vi "Material-Line 3-Normalize.vi"(8 "error in (no error)":errorcluster, 11 "Material-RunTest in":refnum<class "Material-RunTest.lvclass">) -> (0 "error out":errorcluster, 3 "Material-RunTest out":refnum<class "Material-RunTest.lvclass">)   [LabVIEW 2014, in "Material-RunTest.lvclass"]
uses:
  Material-RunTest.lvclass
  <userlib>/_MGI/1D Array/MGI Average/MGI Average (DBL[]).vi
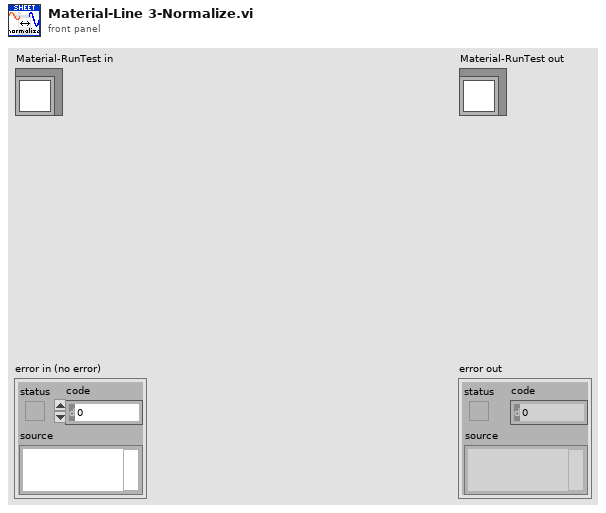
[diagram p1: front panel]
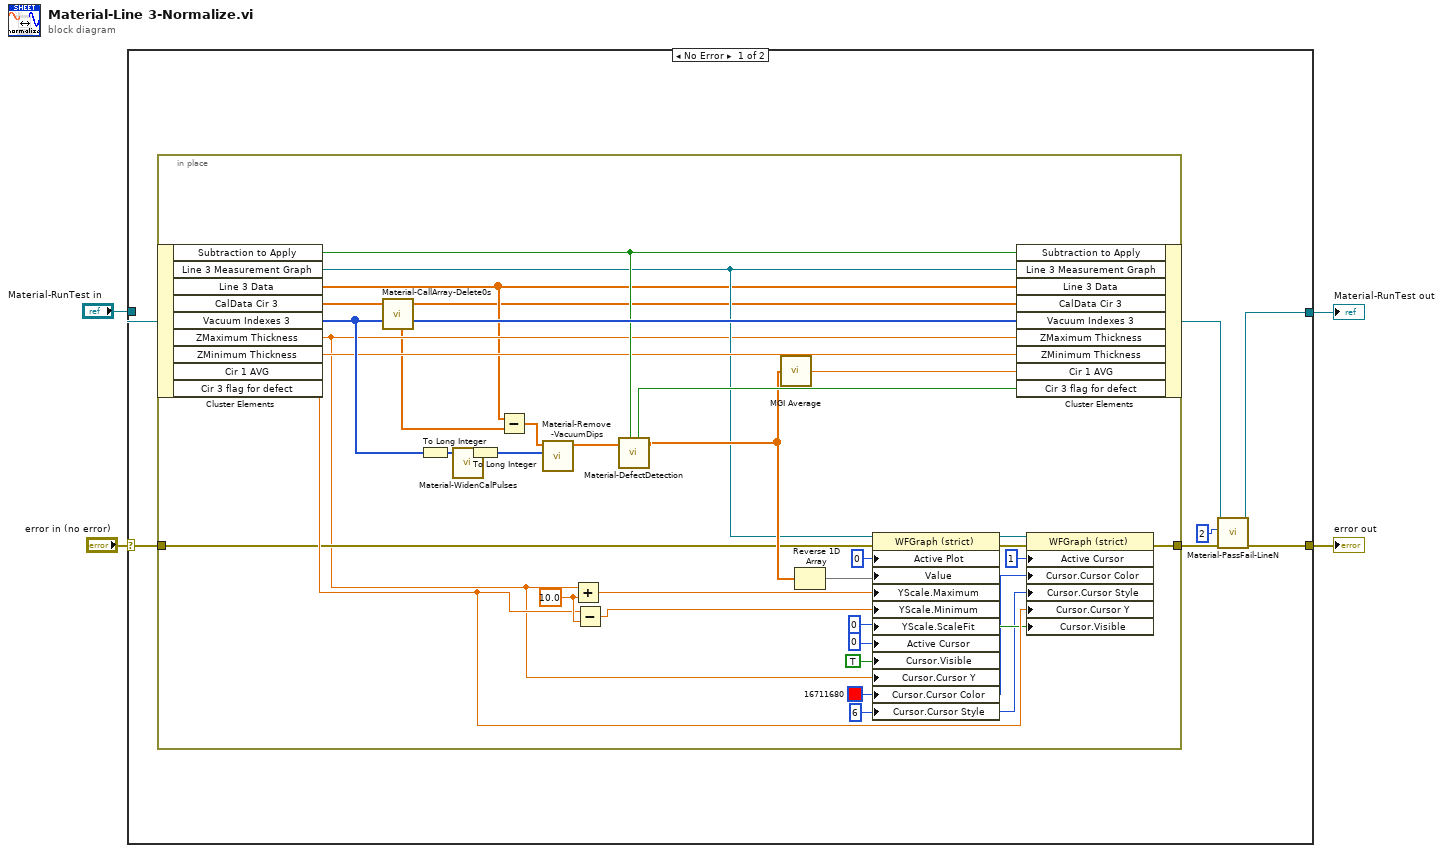
[diagram p0: block diagram]
diagram:
  n1 = case shown="No Error" "error in (no error)" {
    selector: "error in (no error)" -> [w10 w44]
    tunnel: [w7 w44] -> w3
    tunnel: [w5 w43] -> w1
    tunnel: "Material-RunTest in" -> [w11 w43]
    frame No Error {
      n2 = in-place {
        in-place-border: w10 -> [w28]
        in-place-border: [w34] -> w9
        w22 = u32 16711680
        w21 = u8 6 ("Cursor.Cursor Style")
        w23 = TRUE ("Cursor.Visible")
        w38 = 10.0 ("y")
        n3 = in-place-cluster #1(w11) -> ("Subtraction to Apply"=w32:bool, "Line 3 Measurement Graph"=w27:refnum<vi>, "Line 3 Data"=w14:dbl[], "CalData Cir 3"=w13:dbl[], "Vacuum Indexes 3"=w37:i32[], "ZMaximum Thickness"=w20:dbl, "ZMinimum Thickness"=w29:dbl)  [unwired: 2 out]
        n4 = call "Material-CallArray-Delete0s.vi"("CalData Line 3"=w13) -> ("array w/ subset deleted"=w12:dbl[])  [unwired: 8 in]
        n5 = To Long Integer(number=w37) -> (32bit integer=w39:i32[])
        n6 = call "Material-WidenCalPulses.vi"("raw CAL indexes"=w39) -> ("New Indexes"=w41:u32[])  [unwired: 8 in]
        n7 = To Long Integer(number=w41) -> (32bit integer=w42:i32[])
        n8 = Subtract(x=w14, y=w12) -> (x-y=w40:dbl[])
        n9 = call "Material-Remove-VacuumDips.vi"("input array of indexes"=w42, "Input Data"=w40) -> ("Conditioned output"=w33:dbl[])  [unwired: 9 in]
        n10 = Add(x=w20, y=w38) -> (x+y=w18:dbl)
        n11 = Subtract(x=w29, y=w38) -> (x-y=w19:dbl)
        n12 = call "Material-DefectDetection.vi"("Conditioned output"=w33, "Subtraction to Apply"=w32) -> ("Flagged for Defect"=w31:bool, "Array"=w30:dbl[])  [unwired: 6 in]
        n13 = call-poly <userlib>:"MGI Average.vi"("Double[]"=w30) -> ("Average"=w36:dbl)  [unwired: 1 in]
        n14 = Reverse 1D Array(array=w30) -> (reversed array=w17:dbl[])
        n15 = property class="WFGraph (strict)"(reference=w27, error in=w28, "Active Plot"=u32 0, "Value"=w17, "YScale.Maximum"=w18, "YScale.Minimum"=w19, "YScale.ScaleFit"=u8 0 ("Y Scale.Scale Fit"), "Active Cursor"=u32 0, "Cursor.Visible"=w23, "Cursor.Cursor Y"=w20, "Cursor.Cursor Color"=w22, "Cursor.Cursor Style"=w21) -> (reference out=w25:refnum<vi>, error out=w26:errorcluster)
        n16 = in-place-cluster #1("Subtraction to Apply"=w32, "Line 3 Measurement Graph"=w27, "Line 3 Data"=w14, "CalData Cir 3"=w12, "Vacuum Indexes 3"=w37, "ZMaximum Thickness"=w20, "ZMinimum Thickness"=w29, "Cir 1 AVG"=w36, "Cir 3 flag for defect"=w31) -> (w6:refnum<class "Material-RunTest.lvclass">)
        n17 = property class="WFGraph (strict)"(reference=w25, error in=w26, "Active Cursor"=u32 1, "Cursor.Cursor Color"=w22, "Cursor.Cursor Style"=w21, "Cursor.Cursor Y"=w29, "Cursor.Visible"=w23) -> (error out=w34:errorcluster)  [unwired: 1 out]
      }
      n18 = call "Material-PassFail-LineN.vi"("error in (no error)"=w9, "Line?"=2, "Material-RunTest in"=w6) -> ("error out"=w7:errorcluster, "Material-RunTest out"=w5:refnum<class "Material-RunTest.lvclass">)  [unwired: 7 in]
    }
    frame Error {
    }
  }
  "error out" <- w3
  "Material-RunTest out" <- w1
